vi "createCommand.vi"(8 "error in (no error)":errorcluster, 10 "Command":T1, 11 "ICommandFactory in":refnum<class "ICommandFactory.lvclass">) -> (0 "error out":errorcluster, 2 "command":refnum<class "Command.lvclass">, 3 "ICommandFactory out":refnum<class "ICommandFactory.lvclass">)   [LabVIEW 2013, in "ICommandFactory.lvclass"]
uses:
  ICommandFactory.lvclass
  Command/Command.lvclass
  Typedefs/CommandSelector.ctl
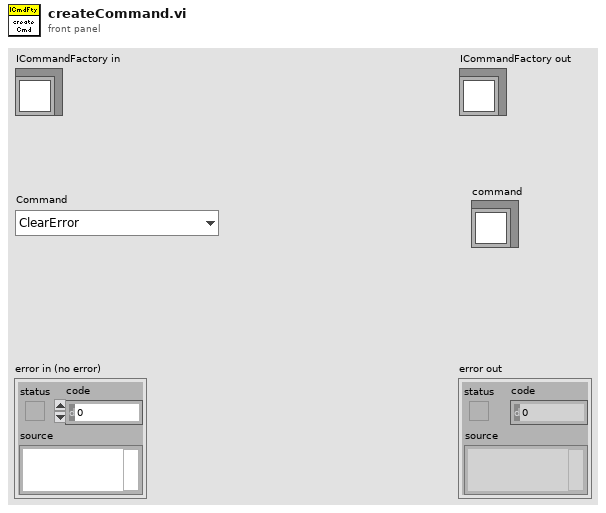
[diagram p1: front panel]
types:
  T1 = typedef "CommandSelector.ctl" = enum16{"ClearError", "Exit", "StandBy", "Start", "SwitchToOnDemandMode", "SwitchToStreamMode", "Update"}
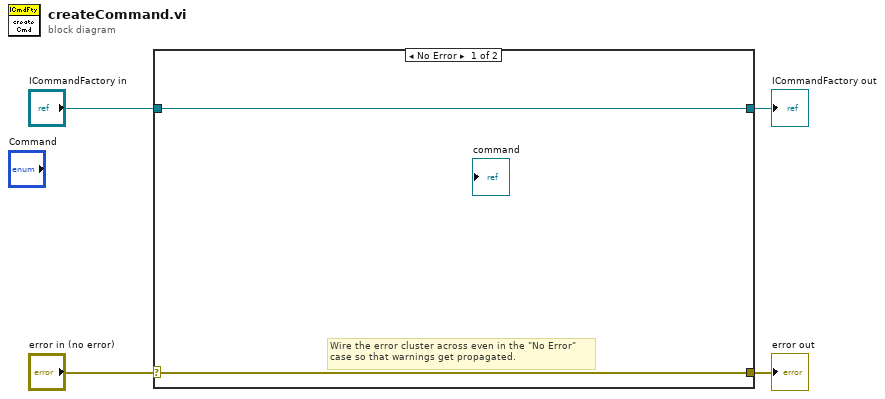
[diagram p0: block diagram]
diagram:
  n1 = case shown="No Error" "error in (no error)" {
    selector: "error in (no error)" -> [w5 w8]
    tunnel: [w5 w8] -> w3
    tunnel: [w6 w7] -> w1
    tunnel: "ICommandFactory in" -> [w6 w7]
    frame No Error {
      # "Wire the error cluster across even in the \"No Error\"\ncase so that warnings get propagated."
    }
    frame Error {
    }
  }
  "error out" <- w3
  "ICommandFactory out" <- w1
